vi "JSONRPC-TestRIP.vi"() -> ()   [LabVIEW 2015]
panel:
  in  "Get 2":string="{\"jsonrpc\":\"2.0\",\"method\":\"get\",\"params\":[\"TestOK\",[\"intout\"]],\"id\":6}"
  in  "Stop":string="{\"jsonrpc\":\"2.0\",\"method\":\"stop\",\"params\":[\"TestOK\"],\"id\":4}"
  in  "Get":string="{\"jsonrpc\":\"2.0\",\"method\":\"get\",\"params\":[\"TestOK\",[\"intout\"]],\"id\":6}"
  in  "Start":string="{\"jsonrpc\":\"2.0\",\"method\":\"start\",\"params\":[\"TestOK\"],\"id\":3}"
  in  "Set":string="{\"jsonrpc\":\"2.0\",\"method\":\"set\",\"params\":[\"TestOK\",[\"intin\"],[2]],\"id\":6}"
  out "Response":string[](array[string])
  # "TestRIP"
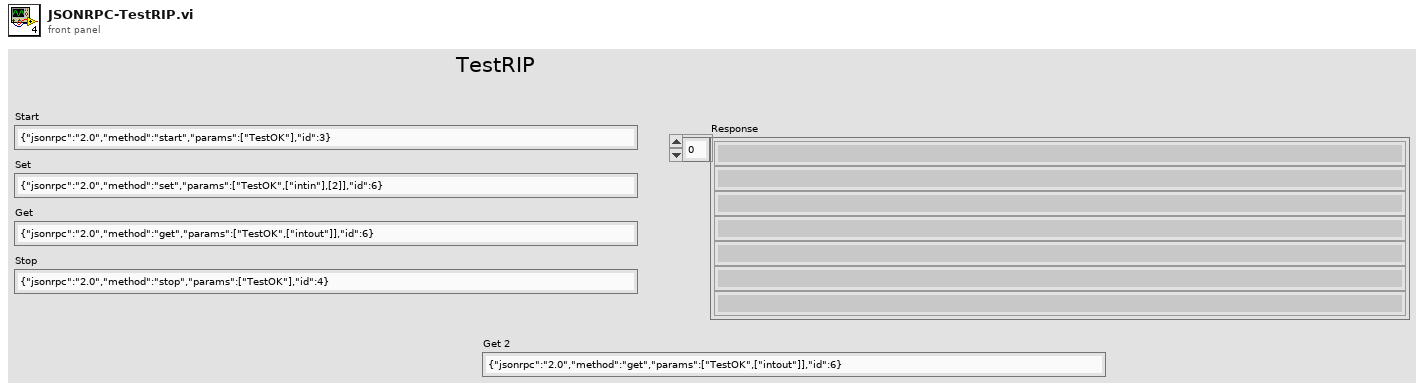
[diagram p1: front panel]
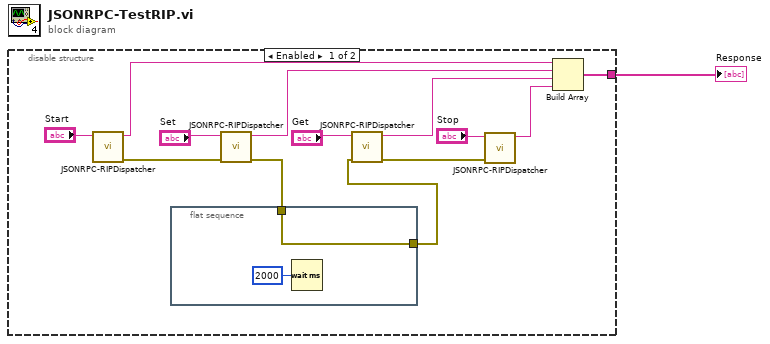
[diagram p0: block diagram]
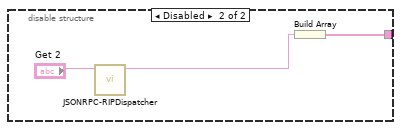
[diagram p2: hidden frame]
diagram:
  n1 = disable-structure shown="Enabled" {
    disable-tunnel: [w4 w18] -> w1
    frame Enabled {
      n2 = call "JSONRPC-RIPDispatcher.vi"("input string"="Start") -> ("error out"=w12:errorcluster, "response"=w8:string)  [unwired: 9 in]
      n3 = flat-sequence {
        tunnel: [w16] -> w2
        tunnel: w3 -> [w16]
        frame #0 {
          n4 = Wait (ms)(milliseconds to wait=u32 2000) -> ()  [unwired: 1 out]
        }
      }
      n5 = call "JSONRPC-RIPDispatcher.vi"("error in"=w12, "input string"="Set") -> ("error out"=w3:errorcluster, "response"=w7:string)  [unwired: 8 in]
      n6 = call "JSONRPC-RIPDispatcher.vi"("error in"=w2, "input string"="Get") -> ("error out"=w10:errorcluster, "response"=w6:string)  [unwired: 8 in]
      n7 = call "JSONRPC-RIPDispatcher.vi"("error in"=w10, "input string"="Stop") -> ("response"=w5:string)  [unwired: 8 in, 1 out]
      n8 = Build Array(w8, w7, w6, w5) -> (w4:string[])
    }
    frame Disabled {
      n9 = call "JSONRPC-RIPDispatcher.vi"("input string"="Get 2") -> ("response"=w17:string)  [unwired: 9 in, 1 out]
      n10 = Build Array(w17) -> (w18:string[])
    }
  }
  "Response" <- w1
